vi "DataRead2D.vi"(0 "Chemin Header":path, 5 "chemin Data":path, 9 "ScanlistIndex":i32, 11 "error in":errorcluster, 12 "XVarParIndex":i32) -> (1 "Header String":string, 2 "2D_Data":dbl[][](array[numeric]), 3 "VarParx":string, 4 "VarPary":string, 6 "X Array":dbl[](array[numeric]), 8 "Y Array 2D":dbl[](array[numeric]), 10 "Y Array":dbl[](array[numeric]), 13 "CurveName":string, 14 "enregistrement(s)":T1={"Entête"="", "Scan list"=[], "NbCourbe"=1, "IndCourbe"=0, "NomDon"=["RTêta;", "X&Y;"], "Session "=0, "Date"="", "Time"="", "VarParams"=[], "UserName"="", "ScanTableSize"=[], "VarPar list"=[], "DescKeyword"=""} caption="ScanParams", 15 "error out":errorcluster)   [LabVIEW 2019]
doc: "Ce VI lit les données contenu dans le fichier de sauvegarde automatique. Ces données correspondent aux valeurs prises lors du dernier balayage. La sauvegarde automatique est effectué après chaque acquisition."
uses:
  Interface Class/ScanParams.ctl
  Interface Class/ScanParamsOld.ctl
  Interface Class/Interface.lvclass
panel:
  in  "YVarParIndex":i32
  out "Data Preview":string[][](array[string])
  out "AllData":dbl[][](array[numeric]) format="%#.8f"
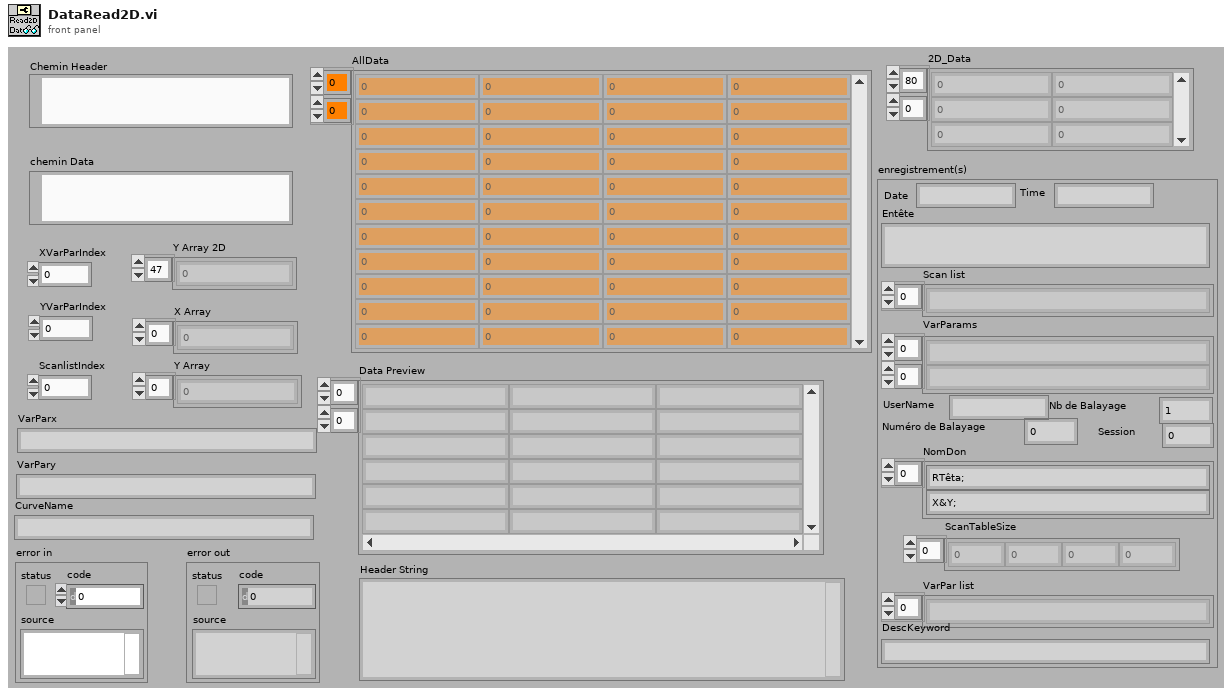
[diagram p1: front panel]
types:
  T1 = typedef "Interface.lvclass/ScanParams.ctl" = cluster{"Entête":string, "Scan list":string[], "NbCourbe":i32, "IndCourbe":i64, "NomDon":string[], "Session ":i32, "Date":string, "Time":string, "VarParams":string[][], "UserName":string, "ScanTableSize":i32[], "VarPar list":string[], "DescKeyword":string}
  T2 = typedef "Interface.lvclass/ScanParamsOld.ctl" = cluster{"Entête":string, "Scan list":string[], "NbCourbe":i32, "IndCourbe":i64, "NomDon":string[], "Session ":i32, "Date":string, "Time":string, "VarParams":string[][], "UserName":string, "ScanTableSize":i32[], "VarPar list":string[]}
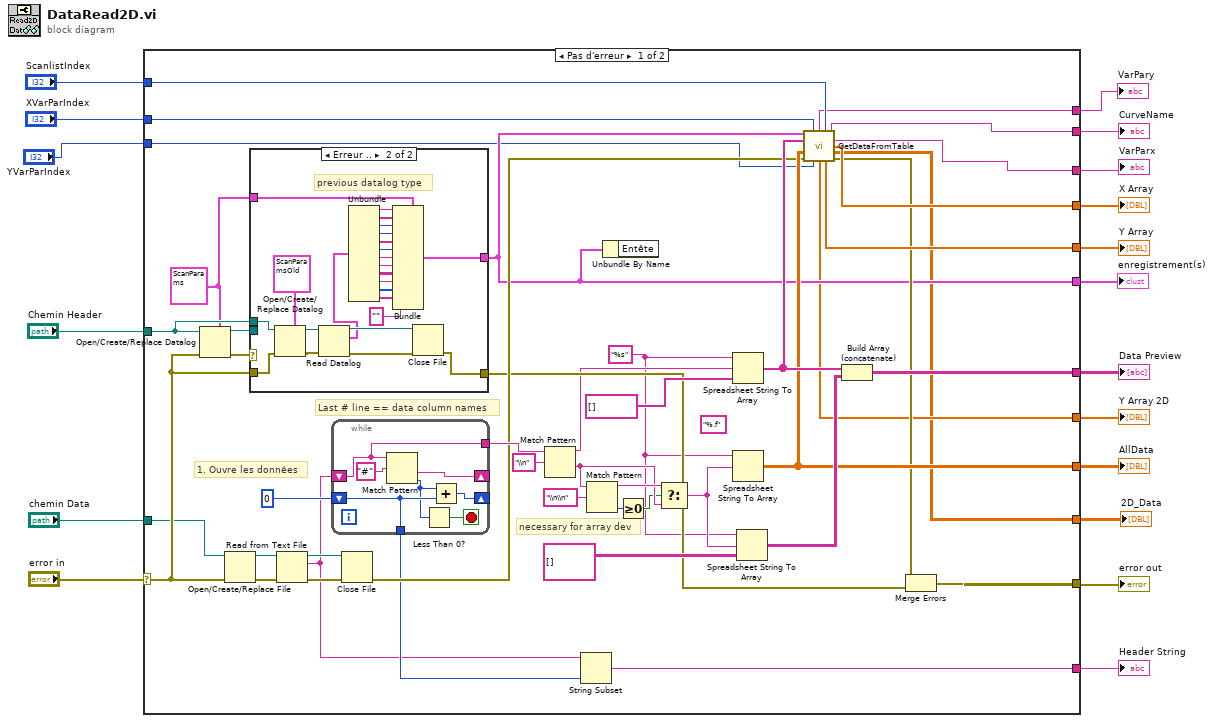
[diagram p0: block diagram]
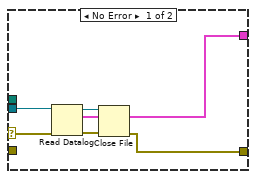
[diagram p2: hidden frame]
diagram:
  n1 = case shown="Pas d'erreur" "error in" {
    selector: "error in" -> [w41 w101]
    tunnel: "chemin Data" -> [w29 _]
    tunnel: [w43 w101] -> w18
    tunnel: [w54 _] -> w15
    tunnel: [w51 _] -> w14
    tunnel: "Chemin Header" -> [w28 _]
    tunnel: "ScanlistIndex" -> [w45 _]
    tunnel: "XVarParIndex" -> [w46 _]
    tunnel: [w50 _] -> w10
    tunnel: [w49 _] -> w9
    tunnel: [w20 _] -> w8
    tunnel: [w21 _] -> w7
    tunnel: [w39 _] -> w6
    tunnel: [w26 _] -> w5
    tunnel: "YVarParIndex" -> [w24 _]
    tunnel: [w23 _] -> w3
    tunnel: [w22 _] -> w2
    tunnel: [w19 _] -> w1
    frame No Error {
      (unwired) "%.f" ("séparateur (Tabulation)")
      w27 = T1 {"Entête"="", "Scan list"=[], "NbCourbe"=1, "IndCourbe"=1, "NomDon"=["RTêta;", "X&Y;"], "Session "=0, "Date"="", "Time"="", "VarParams"=[], "UserName"="", "ScanTableSize"=[], "VarPar list"=[], "DescKeyword"=""} ("ScanParams")
      w25 = "%s" ("chaîne de format")
      # "necessary for array dev"
      # "Last # line == data column names"
      # "1. Ouvre les données"
      n2 = Open/Create/Replace Datalog(5:w27, 8:w41, 11:w28) -> (0:w44:errorcluster, 3:w57:refnum<k1>)  [unwired: 3 in, 1 out]
      n3 = Open/Create/Replace File(file path (use dialog)=w29, error in=w41) -> (refnum out=w63:refnum<file>, error out=w62:errorcluster)  [unwired: 4 in, 1 out]
      n4 = case shown="Erreur .." w44 {
        selector: w44 -> [w66 _]
        tunnel: w57 -> [w69 _]
        tunnel: [w64 w72] -> w26
        tunnel: w28 -> [_ w88]
        tunnel: [w65 w73] -> w42
        tunnel: w41 -> [_ w71]
        tunnel: w27 -> [_ w70]
        frame No Error {
          n5 = Read Datalog(4:w66, 7:w69) -> (0:w68:errorcluster, 2:w64:T1, 3:w67:refnum<k1>)  [unwired: 1 in]
          n6 = Close File(refnum=w67, error in=w68) -> (error out=w65:errorcluster)  [unwired: 1 out]
        }
        frame Error {
          # "previous datalog type"
          n7 = Open/Create/Replace Datalog(5:T2 {"Entête"="", "Scan list"=[], "NbCourbe"=1, "IndCourbe"=1, "NomDon"=["RTêta;", "X&Y;"], "Session "=0, "Date"="", "Time"="", "VarParams"=[], "UserName"="", "ScanTableSize"=[], "VarPar list"=[]} ("ScanParams"), 8:w71, 11:w88) -> (0:w90:errorcluster, 3:w91:refnum<k1>)  [unwired: 3 in, 1 out]
          n8 = Read Datalog(4:w90, 7:w91) -> (0:w93:errorcluster, 2:w87:T2, 3:w92:refnum<k1>)  [unwired: 1 in]
          n9 = Unbundle(w87) -> ("Entête"=w86:string, "Scan list"=w85:string[], "NbCourbe"=w84:i32, "IndCourbe"=w83:i64, "NomDon"=w82:string[], "Session"=w81:i32, "Date"=w80:string, "Time"=w79:string, "VarParams"=w78:string[][], "UserName"=w77:string, "ScanTableSize"=w76:i32[], "VarPar list"=w75:string[])
          n10 = Bundle(cluster=w70, "Entête"=w86, "Scan list"=w85, "NbCourbe"=w84, "IndCourbe"=w83, "NomDon"=w82, "Session"=w81, "Date"=w80, "Time"=w79, "VarParams"=w78, "UserName"=w77, "ScanTableSize"=w76, "VarPar list"=w75, "DescKeyword"="") -> (w72:T1)
          n11 = Close File(refnum=w92, error in=w93) -> (error out=w73:errorcluster)  [unwired: 1 out]
        }
      }
      n12 = Read from Text File(file (use dialog)=w63, error in=w62) -> (refnum out=w60:refnum<file>, text=w30:string, error out=w61:errorcluster)  [unwired: 2 in, 1 out]
      n13 = while {
        shift-right: [w99] -> _
        shift-left: w30 -> [w97]
        tunnel: [w97] -> w59
        shift-right: [w94] -> _
        shift-left: 0 ("offset past match") -> [w96]
        tunnel: [w96] -> w38
        stop <- w98 stop-if-true
        n14 = Match Pattern(string=w97, regular expression="#" ("expression régulière")) -> (after substring=w99:string, offset past match=w95:i32)  [unwired: 1 in, 2 out]
        n15 = Less Than 0?(x=w95) -> (x < 0?=w98:bool)
        n16 = Add(x=w95, y=w96) -> (x+y=w94:i32)
      }
      n17 = Close File(refnum=w60, error in=w61) -> (error out=w47:errorcluster)  [unwired: 1 out]
      n18 = Match Pattern(string=w59, regular expression="\\n" ("expression régulière")) -> (before substring=w31:string, after substring=w34:string)  [unwired: 1 in, 2 out]
      n19 = String Subset(string=w30, length (rest)=w38) -> (substring=w39:string)  [unwired: 1 in]
      n20 = Match Pattern(string=w34, regular expression="\\n\\n" ("expression régulière")) -> (before substring=w36:string, offset past match=w32:i32)  [unwired: 1 in, 2 out]
      n21 = Unbundle By Name(w26) -> ()  [unwired: 1 out]
      n22 = Greater Or Equal To 0?(x=w32) -> (x >= 0?=w33:bool)
      n23 = Select(t=w36, s=w33, f=w34) -> (s? t:f=w35:string)
      n24 = Spreadsheet String To Array(format string=w25, spreadsheet string=w31, array type (2D Dbl)=string[] []) -> (array=w52:string[])  [unwired: 1 in]
      n25 = Spreadsheet String To Array(format string=w25, spreadsheet string=w35) -> (array=w51:dbl[][])  [unwired: 2 in]
      n26 = Spreadsheet String To Array(format string=w25, spreadsheet string=w35, array type (2D Dbl)=string[][] []) -> (array=w55:string[][])  [unwired: 1 in]
      n27 = call "GetDataFromTable.vi"("DataRecord"=w26, "XVarParIndex"=w46, "ScanlistIndex"=w45, "FilesColName"=w52, "AllDataIn"=w51, "error in"=w47, "YVarParIndex"=w24) -> ("Y_VarPar"=w19:string, "CurveName"=w21:string, "VarPar"=w20:string, "X Array"=w49:dbl[], "2D_Data"=w22:dbl[][], "Y Array"=w23:dbl[], "Data Array"=w50:dbl[], "error out"=w48:errorcluster)  [unwired: 1 in]
      n28 = Build Array (concatenate)(w52, w55) -> (w54:string[][])
      n29 = Merge Errors(w48, w42) -> (w43:errorcluster)
    }
    frame Error {
    }
  }
  "error out" <- w18
  "Data Preview" <- w15
  "AllData" <- w14
  "Y Array" <- w10
  "X Array" <- w9
  "VarParx" <- w8
  "CurveName" <- w7
  "Header String" <- w6
  "enregistrement(s)" <- w5
  "VarPary" <- w1
  "Y Array 2D" <- w3
  "2D_Data" <- w2
